vi "FSN.vi"(0 "System no.":i32=1 min=1 step=1, 1 "Board":i32=1 min=1 max=5 step=1, 2 "Axes to scan":string[](array[string]), 3 "Scan range":dbl[](array[numeric]) format="%.6f", 4 "No.of digits":i16=4, 5 "error in":errorcluster, 6 "Treshold level":dbl=1.0 format="%.3f", 7 "D":dbl=1.0, 8 "R":dbl, 9 "C":dbl, 10 "Use #7 polling?":bool, 11 "Timeout (s)":dbl=300.0 min=1.0 max=4.0 step=1.0 format="%.2f", 12 "Stop refnum":refnum<vi>) -> (14 "Scan successful?":bool, 19 "error out":errorcluster)   [LabVIEW 2026]
doc: "Performs a 1D scan following a trajectory described by the given parameters, waits until scan is ready (using #7 polling if checked) and indicates whether scan was successful or not. Timeout is only valid if Use #7 polling is FALSE. If Refnum stop or Local stop is TRUE, VI sends #24 and stops. See system manual for further details.\n\nF-206: Use #7 polling = FALSE, Axes to scan can be a subset of (X,Y,Z,U,V,W). Scan cannot be stopped. Only for GCS syntax version = GCS 1.0 (check with CSV?.vi. If CSV?.vi is not supported, syntax version is GCS 1.0).\n\nC-887, M-8X0: Use #7 polling = FALSE, Axes to scan can be a subset of (X,Y,Z,U,V,W). Scan cannot be stopped. Only for GCS syntax version = GCS 1.0 (check with CSV?.vi. If CSV?.vi is not supported, syntax version is GCS 1.0)."
panel:
  in  "Local stop":bool
  # "Performs a 1D scan following a trajectory decribed by the given parameters, waits \nuntil scan is ready (using #7 polling if checked) and indicates whether scan was \nsuccessful or not. \"Timeout\" is only valid if \"Use #7 polling\" is FALSE. If Stop refnum\nor Local stop is TRUE, VI sends #24 and stops. See system manual for further \ndetails."
  # "Scan range:"
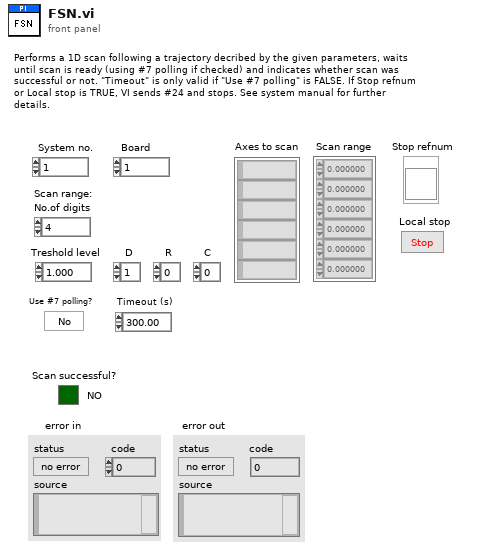
[diagram p1: front panel]
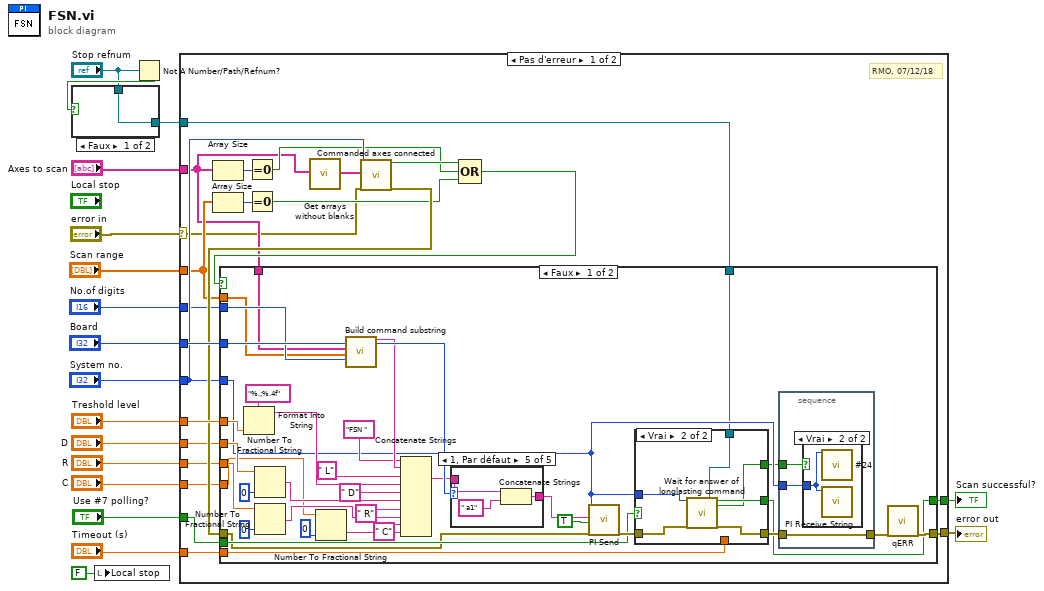
[diagram p0: block diagram]
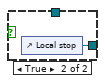
[diagram p2: hidden frame]
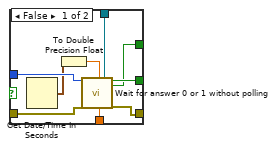
[diagram p4: hidden frame]
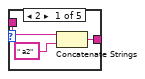
[diagram p5: hidden frame]
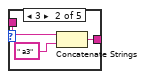
[diagram p6: hidden frame]
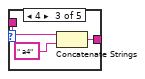
[diagram p7: hidden frame]
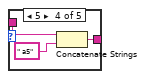
[diagram p8: hidden frame]
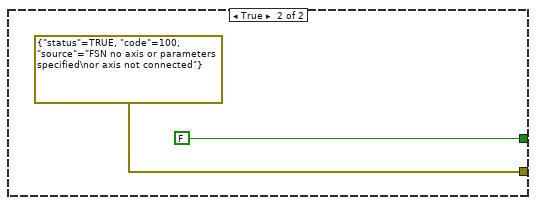
[diagram p9: hidden frame]
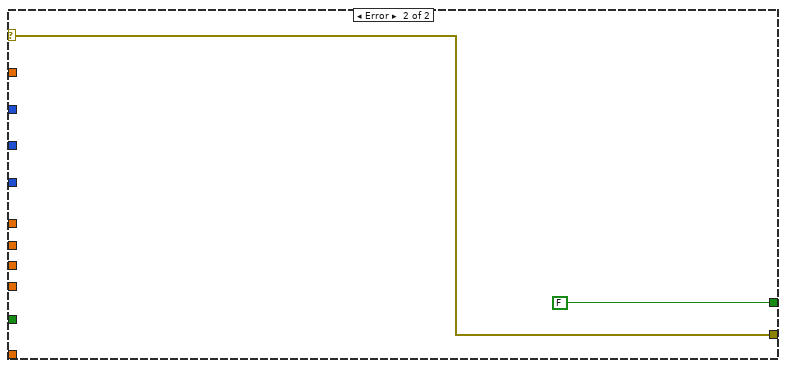
[diagram p10: hidden frame]
diagram:
  n1 = local write "Local stop"(FALSE ("Local stop")) -> ()
  n2 = Not A Number/Path/Refnum?(number/path/refnum="Stop refnum") -> (NaN/Path/Refnum?=w4:bool)
  n3 = case shown="Faux" w4 {
    tunnel: [w19 w20] -> w2
    tunnel: "Stop refnum" -> [w19 _]
    frame False {
    }
    frame True {
      n4 = control-ref of="Local stop"() -> (w20:refnum<vi>)
    }
  }
  n5 = case shown="Pas d'erreur" "error in" {
    selector: "error in" -> [w21 w116]
    tunnel: "System no." -> [w35 _]
    tunnel: [w40 w116] -> w17
    tunnel: [w39 FALSE] -> w16
    tunnel: "Board" -> [w43 _]
    tunnel: "Treshold level" -> [w42 _]
    tunnel: "Use #7 polling?" -> [w38 _]
    tunnel: "Timeout (s)" -> [w37 _]
    tunnel: "Axes to scan" -> [w23 _]
    tunnel: "D" -> [w34 _]
    tunnel: "R" -> [w33 _]
    tunnel: "C" -> [w32 _]
    tunnel: "No.of digits" -> [w29 _]
    tunnel: "Scan range" -> [w27 _]
    tunnel: w2 -> [w22 _]
    frame No Error {
      # "RMO, 07/12/18"
      n6 = Array Size(array=w23) -> (size(s)=w30:i32)
      n7 = Array Size(array=w27) -> (size(s)=w28:i32)
      n8 = Equal To 0?(x=w30) -> (x = 0?=w25:bool)
      n9 = Equal To 0?(x=w28) -> (x = 0?=w24:bool)
      n10 = call "Get arrays without blanks.vi"("String array in"=w23) -> ("String array out"=w36:string[])  [unwired: 2 in, 16 out]
      n11 = call "Commanded axes connected.vi"("System no."=w35, "Commanded axes"=w36, "error in"=w21) -> ("Controller error"=w26:bool, "error out"=w41:errorcluster)  [unwired: 15 out]
      n12 = Compound Arithmetic op=OR(w26, w25, w24) -> (w31:bool)
      n13 = case shown="Faux" w31 {
        tunnel: w43 -> [w79 _]
        tunnel: w42 -> [w71 _]
        tunnel: w41 -> [w62 _]
        tunnel: w35 -> [w46 _]
        tunnel: [w48 errorcluster {"status"=TRUE, "code"=100, "source"="FSN no axis or parameters specified\nor axis not connected"} ("error out")] -> w40
        tunnel: [w47 FALSE] -> w39
        tunnel: w38 -> [w74 _]
        tunnel: w37 -> [w73 _]
        tunnel: w23 -> [w53 _]
        tunnel: w34 -> [w64 _]
        tunnel: w33 -> [w60 _]
        tunnel: w32 -> [w57 _]
        tunnel: w29 -> [w55 _]
        tunnel: w27 -> [w54 _]
        tunnel: w22 -> [w45 _]
        frame False {
          n14 = Format Into String(format string="%.;%.4f" ("Format String"), w71) -> (resulting string=w69:string)  [unwired: 2 in, 1 out]
          n15 = Number To Fractional String(number=w64, precision (6)=i16 0) -> (F-format string=w63:string)  [unwired: 2 out]
          n16 = Number To Fractional String(number=w60, precision (6)=i16 0) -> (F-format string=w59:string)  [unwired: 2 out]
          n17 = Number To Fractional String(number=w57, precision (6)=i16 0) -> (F-format string=w56:string)  [unwired: 2 out]
          n18 = call "Build command substring.vi"("Affected axes"=w53, "Parameters"=w54, "No. of digits"=w55) -> ("Command substring"=w52:string)  [unwired: 4 in, 12 out]
          n19 = Concatenate Strings("FSN ", w52, " L", w69, " D", w63, " R", w59, " C", w56) -> (w78:string)
          n20 = case shown="1, Par défaut" w79 {
            tunnel: w78 -> [w101 w104 w107 w110 w113]
            tunnel: [w99 w102 w105 w108 w111] -> w77
            frame 2 {
              n21 = Concatenate Strings(w101, " a2" ("Substring")) -> (w99:string)
            }
            frame 3 {
              n22 = Concatenate Strings(w104, " a3" ("Substring")) -> (w102:string)
            }
            frame 4 {
              n23 = Concatenate Strings(w107, " a4" ("Substring")) -> (w105:string)
            }
            frame 5 {
              n24 = Concatenate Strings(w110, " a5" ("Substring")) -> (w108:string)
            }
            frame 1, Default {
              n25 = Concatenate Strings(w113, " a1" ("Substring")) -> (w111:string)
            }
          }
          n26 = call "PI Send.vi"("System no."=w46, "String to send"=w77, "Attach termination char.?"=TRUE ("Attach Linefeed?"), "error in"=w62) -> ("error out"=w75:errorcluster)  [unwired: 2 in, 13 out]
          n27 = case shown="Vrai" w74 {
            tunnel: w46 -> [w92 w98]
            tunnel: w75 -> [w91 w97]
            tunnel: [w90 w96] -> w49
            tunnel: [w89 w95] -> w47
            tunnel: w73 -> [w87 _]
            tunnel: w45 -> [w86 w94]
            tunnel: [w85 w93] -> w44
            frame False {
              n28 = Get Date/Time In Seconds() -> (seconds since 1Jan1904=w84:timestamp)
              n29 = To Double Precision Float(number=w84) -> (double precision float=w88:dbl)
              n30 = call "Wait for answer 0 or 1 without polling.vi"("System no."=w92, "error in"=w91, "Start time"=w88, "Timeout (s)"=w87, "Stop refnum"=w86) -> ("Scan successful?"=w89:bool, "Stopped"=w85:bool, "error out"=w90:errorcluster)  [unwired: 12 out]
            }
            frame True {
              n31 = call "Wait for answer of longlasting command.vi"("System no."=w98, "error in"=w97, "Stop refnum"=w94) -> ("Answer"=w95:bool, "Stopped"=w93:bool, "error out"=w96:errorcluster)  [unwired: 14 out]
            }
          }
          n32 = stacked-sequence {
            tunnel: w46 -> [w82]
            tunnel: [w81] -> w50
            tunnel: w49 -> [w81]
            tunnel: w44 -> [w80]
            frame #0 {
              n33 = case shown="Vrai" w80 {
                tunnel: w82 -> [_ w83]
                frame False {
                }
                frame True {
                  n34 = call "#24.vi"("System no."=w83) -> ()  [unwired: 1 in, 18 out]
                  n35 = call "PI Receive String.vi"("System no."=w83) -> ()  [unwired: 2 in, 17 out]
                }
              }
            }
          }
          n36 = call "qERR.vi"("error in"=w50) -> ("error out"=w48:errorcluster)  [unwired: 1 in, 17 out]
        }
        frame True {
        }
      }
    }
    frame Error {
    }
  }
  "error out" <- w17
  "Scan successful?" <- w16
